vi "TestBaxter.vi"() -> ()   [LabVIEW 2012]
uses:
  <userlib>/rosforlv/ROS/Code/SubVIs/BaxterSide.ctl
  <userlib>/rosforlv/ROS/Code/SubVIs/BaxterCamera.ctl
panel:
  in  "Camera Settings":T2={"Camera"=enum."left_hand_camera", "FPS"=20.0, "Camera Controls"=[], "Resolution"=enum."(320, 200)"}
  out "new picture":picture
  in  "Get Image":bool
  out "error out":errorcluster
  in  "Set Gripper":bool
  in  "Nod":bool
  in  "stop":bool
  in  "Gripper Position":sgl=100.0 min=0 max=100
  in  "Gripper Side":T3
  in  "Green Level":sgl
  in  "Red Level":sgl
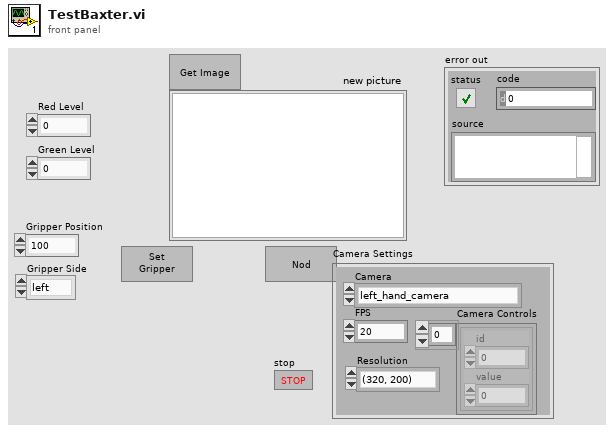
[diagram p1: front panel]
types:
  T1 = typedef "BaxterCamera.ctl" = enum16{"left_hand_camera", "right_hand_camera", "head_camera"}
  T2 = cluster{"Camera":T1, "FPS":sgl, "Camera Controls":cluster{"id":i32, "value":i32}[], "Resolution":enum16{"(1280, 800)", "(960, 600)", "(640, 400)", "(480, 300)", "(384, 240)", "(320, 200)"}}
  T3 = typedef "BaxterSide.ctl" = enum16{"left", "right"}
  T4 = typedef "QT_Image.ctl" = cluster{"Width":i32, "Height":i32, "Depth":i32, "data":u8[], "Compressed data":u8[], "Color table":u32[], "Duration":i32, "Options":i32, "Timestamp":i32, "ID":i32, "Reserved":i32, "Dialogs":u32}
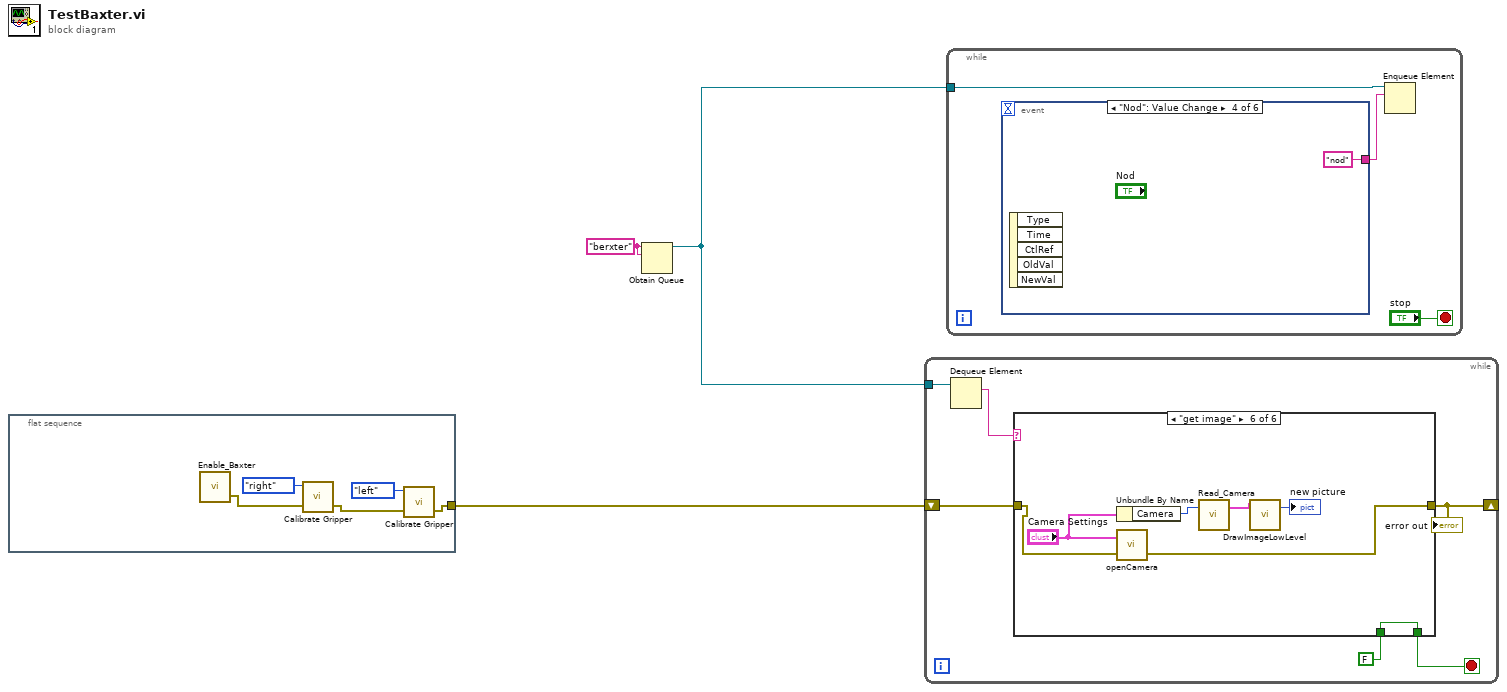
[diagram p0: block diagram]
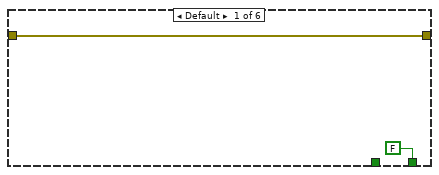
[diagram p2: hidden frame]
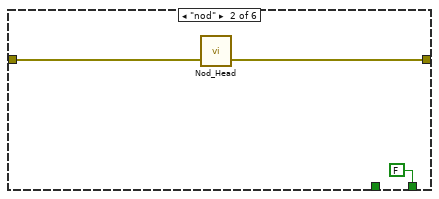
[diagram p3: hidden frame]
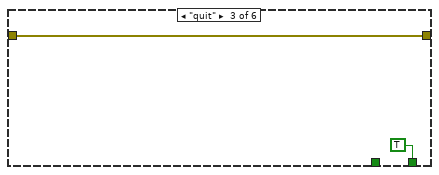
[diagram p4: hidden frame]
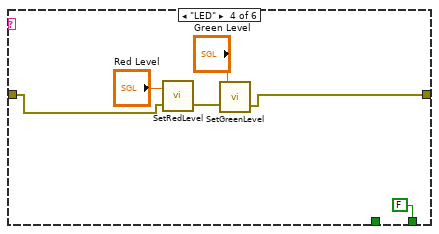
[diagram p5: hidden frame]
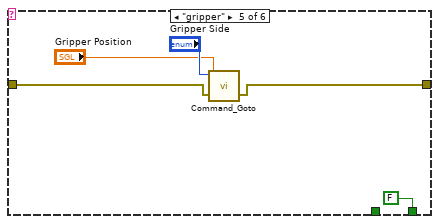
[diagram p6: hidden frame]
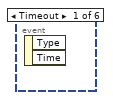
[diagram p7: hidden frame]
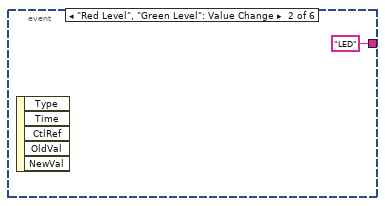
[diagram p8: hidden frame]
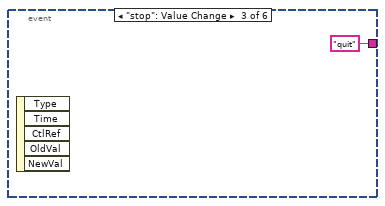
[diagram p9: hidden frame]
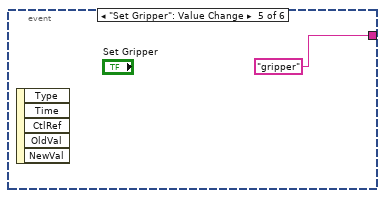
[diagram p10: hidden frame]
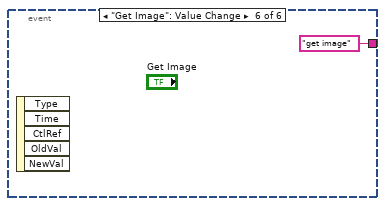
[diagram p11: hidden frame]
diagram:
  w2 = "berxter" ("name (unnamed)")
  n1 = flat-sequence {
    tunnel: [w8] -> w1
    frame #0 {
      n2 = call <userlib>:"Enable_Baxter.vi"() -> ("error out"=w4:errorcluster)  [unwired: 4 in]
      n3 = call <userlib>:"Calibrate Gripper.vi"("Side"=BaxterSide."right", "error in"=w4) -> ("error out"=w5:errorcluster)  [unwired: 4 in]
      n4 = call <userlib>:"Calibrate Gripper.vi"("Side"=BaxterSide."left", "error in"=w5) -> ("error out"=w8:errorcluster)  [unwired: 4 in]
    }
  }
  n5 = Obtain Queue(name (unnamed)=w2, element data type=w2) -> (queue out=w3:refnum<queue>)  [unwired: 3 in, 2 out]
  n6 = while {
    tunnel: w3 -> [w14]
    shift-right: [w12] -> _
    shift-left: w1 -> [w11]
    stop <- w10 stop-if-true
    n7 = Dequeue Element(queue=w14) -> (element=w13:string)  [unwired: 2 in, 3 out]
    n8 = case shown="\"get image\"" w13 {
      tunnel: [w16 w19 w20 w23 w29 w33] -> w12
      tunnel: w11 -> [w16 w18 w20 w24 w30 w34]
      tunnel: [FALSE FALSE TRUE FALSE FALSE w37] -> w10
      tunnel: FALSE -> [_ _ _ _ _ w37]
      frame Default {
      }
      frame "nod" {
        n9 = call <userlib>:"Nod_Head.vi"("error in"=w18) -> ("error out"=w19:errorcluster)  [unwired: 3 in]
      }
      frame "quit" {
      }
      frame "LED" {
        n10 = call <userlib>:"SetRedLevel.vi"("error in"=w24, "Numeric"="Red Level") -> ("error out"=w27:errorcluster)  [unwired: 1 in]
        n11 = call <userlib>:"SetGreenLevel.vi"("error in"=w27, "Numeric"="Green Level") -> ("error out"=w23:errorcluster)  [unwired: 1 in]
      }
      frame "gripper" {
        n12 = call <userlib>:"Command_Goto.vi"("Side"="Gripper Side", "Desired Position"="Gripper Position", "error in"=w30) -> ("error out"=w29:errorcluster)  [unwired: 3 in]
      }
      frame "get image" {
        n13 = Unbundle By Name("Camera Settings") -> ("Camera"=w35:T1)
        n14 = call <userlib>:"openCamera.vi"("error in"=w34, "Camera Settings"="Camera Settings") -> ("error out"=w33:errorcluster)  [unwired: 1 in, 1 out]
        n15 = call <userlib>:"Read_Camera.vi"("Camera"=w35) -> ("image out"=w39:T4)  [unwired: 2 in, 1 out]
        n16 = call <userlib>:"DrawImageLowLevel.vi"("Image"=w39) -> ("new picture"=→"new picture":picture)  [unwired: 4 in, 1 out]
      }
    }
    "error out" <- w12
  }
  n17 = while {
    tunnel: w3 -> [w42]
    stop <- "stop" stop-if-true
    n18 = event shown="[3] \"Nod\": Value Change" {
      selector: _ -> [_ _ _ _ _ _]
      dyn-events: _ -> [_ _ _ _ _ _]
      timeout: _ -> [_ _ _ _ _ _]
      tunnel: [_ "LED" ("element") "quit" ("element") "nod" ("element") "gripper" ("element") "get image" ("element")] -> w40
      event Timeout {
        n19 = event-data() -> ()  [unwired: 1 in, 2 out]
      }
      event "Red Level", "Green Level": Value Change {
        n20 = event-data() -> ()  [unwired: 1 in, 5 out]
      }
      event "stop": Value Change {
        n21 = event-data() -> ()  [unwired: 1 in, 5 out]
      }
      event "Nod": Value Change {
        n22 = event-data() -> ()  [unwired: 1 in, 5 out]
      }
      event "Set Gripper": Value Change {
        n23 = event-data() -> ()  [unwired: 1 in, 5 out]
      }
      event "Get Image": Value Change {
        n24 = event-data() -> ()  [unwired: 1 in, 5 out]
      }
    }
    n25 = Enqueue Element(queue=w42, element=w40) -> ()  [unwired: 2 in, 3 out]
  }
